vi "Save_Pointer_Offset.vi"(1 "Values":dbl[](array[numeric]) format="%.4f", 3 "Mode":T1(ring)) -> (0 "Values Out":dbl[](array[numeric]) format="%.2f")   [LabVIEW 2010]
uses:
  Globals/Constants_global.vi
  Globals/Trav_pos_global.vi
panel:
  # "X                                  Y                          Z"
  # "X                    Y                 Z"
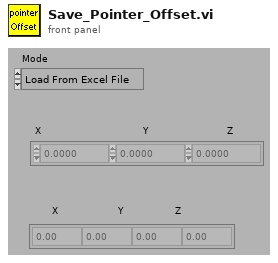
[diagram p1: front panel]
types:
  T1 = enum16{"Load From Excel File", "Save to Excel File"}
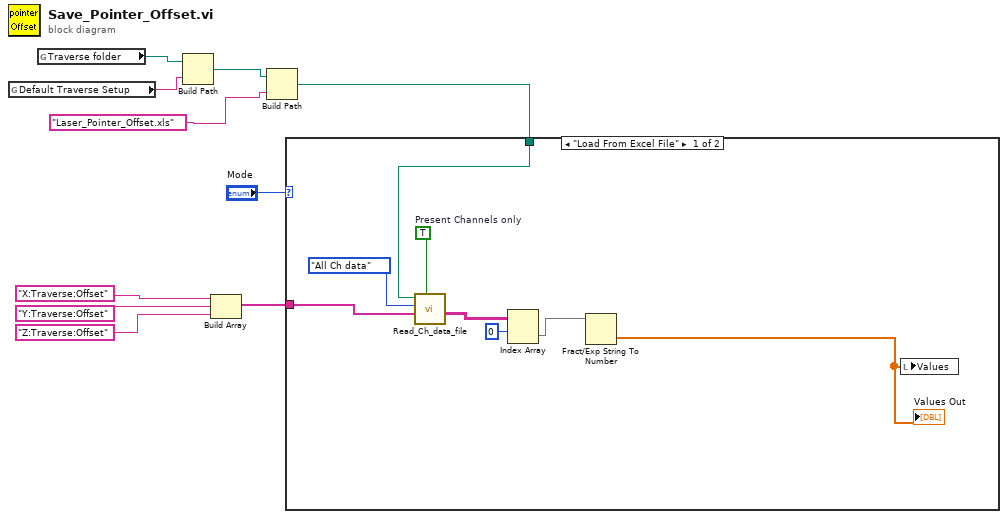
[diagram p0: block diagram]
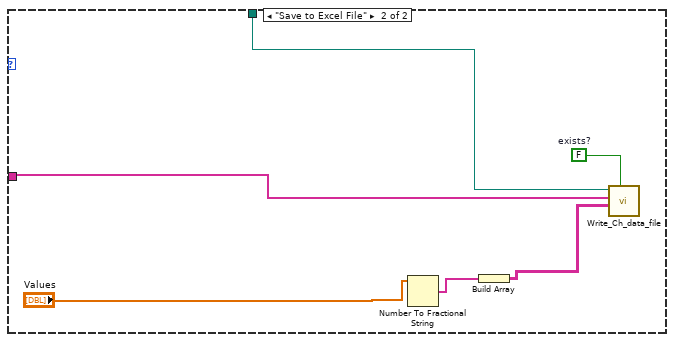
[diagram p2: hidden frame]
diagram:
  n1 = global read "Trav_pos_global.vi" "Default Traverse Setup"() -> (w2:string)
  n2 = global read "Constants_global.vi" "Traverse folder"() -> (w7:path)
  n3 = Build Path(base path=w7, name or relative path=w2) -> (appended path=w4:path)
  n4 = Build Array("X:Traverse:Offset", "Y:Traverse:Offset", "Z:Traverse:Offset") -> (w6:string[])
  n5 = Build Path(base path=w4, name or relative path="Laser_Pointer_Offset.xls" ("Substring")) -> (appended path=w3:path)
  n6 = case shown="\"Load From Excel File\"" "Mode" {
    tunnel: w6 -> [w16 w22]
    tunnel: w3 -> [w15 w23]
    frame "Load From Excel File" {
      w18 = TRUE  # Present Channels only
      n7 = call "Read_Ch_data_file.vi"("Present Channels only"=w18, "Present Channels"=w16, "Output"=enum16{"All Ch data", "The last few rows"}."All Ch data", "Filename"=w15) -> ("Channel Values"=w14:string[][])  [unwired: 1 in, 4 out]
      n8 = Index Array(array=w14, index (row)=0) -> (element=w12:string[])  [unwired: 1 in]
      n9 = Fract/Exp String To Number(string=w12) -> (number=w11:dbl[])  [unwired: 3 in, 1 out]
      "Values Out" <- w11
      n10 = local write "Values"(w11) -> ()
    }
    frame "Save to Excel File" {
      w24 = FALSE  # exists?
      n11 = Number To Fractional String(number="Values") -> (F-format string=w20:string[])  [unwired: 3 in]
      n12 = Build Array(w20) -> (w19:string[][])
      n13 = call "Write_Ch_data_file.vi"("exists?"=w24, "Channel Values"=w19, "Channel names"=w22, "Filename"=w23) -> ()  [unwired: 8 in]
    }
  }
